vi "SA_fgv.vi"(6 "value":u32=35, 7 "command":T1=enum."set system index") -> (0 "rotation channel":u32, 1 "y channel":u32, 2 "x channel":u32, 3 "system index":u32)   [LabVIEW 2016]
uses:
  sa commands.ctl
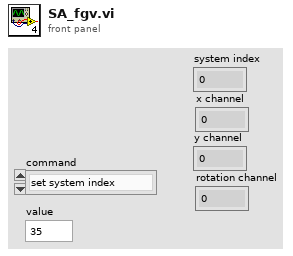
[diagram p1: front panel]
types:
  T1 = typedef "sa commands.ctl" = enum16{"read all", "set system index", "set x channel", "set y channel", "set rotation channel"}
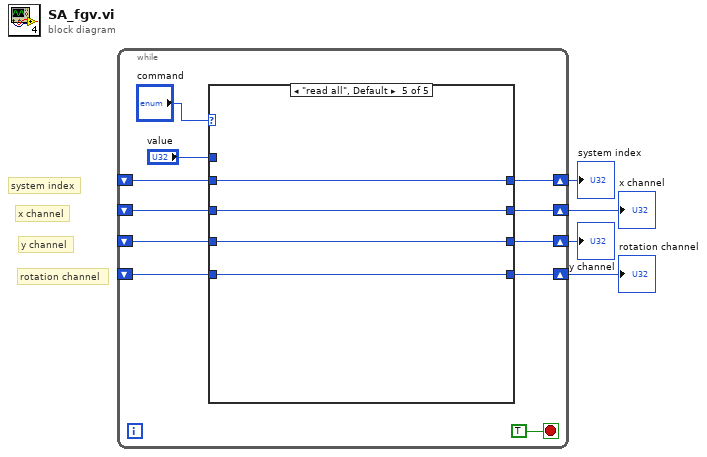
[diagram p0: block diagram]
diagram:
  # "rotation channel"
  # "y channel"
  # "x channel"
  # "system index"
  n1 = while {
    shift-right: [w13] -> w4
    shift-left: _ -> [w12]
    shift-right: [w11] -> w3
    shift-left: _ -> [w8]
    shift-right: [w10] -> w2
    shift-left: _ -> [w7]
    shift-right: [w9] -> w1
    shift-left: _ -> [w6]
    stop <- TRUE stop-if-true
    n2 = case shown="\"read all\", Default" "command" {
      tunnel: [w19 w22 w25 w28 w35] -> w13
      tunnel: w12 -> [_ w22 w25 w28 w35]
      tunnel: [w18 w23 w26 w29 w34] -> w11
      tunnel: [w17 w21 w27 w30 w33] -> w10
      tunnel: [w16 w20 w24 w31 w32] -> w9
      tunnel: w8 -> [w18 _ w26 w29 w34]
      tunnel: w7 -> [w17 w21 _ w30 w33]
      tunnel: w6 -> [w16 w20 w24 _ w32]
      tunnel: "value" -> [w19 w23 w27 w31 _]
      frame "set system index" {
      }
      frame "set x channel" {
      }
      frame "set y channel" {
      }
      frame "set rotation channel" {
      }
      frame "read all", Default {
      }
    }
  }
  "system index" <- w4
  "x channel" <- w3
  "y channel" <- w2
  "rotation channel" <- w1
